vi "BIT2DEC Calculator.vi"() -> ()   [LabVIEW 2022 SP3]
panel:
  out "DEC Data(Result)":dbl
  out "Mantissa Data":dbl
  out "Exponential Data":dbl
  out "Sign Data":dbl
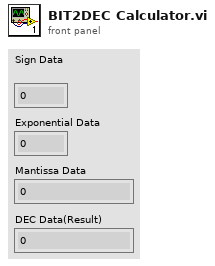
[diagram p1: front panel]
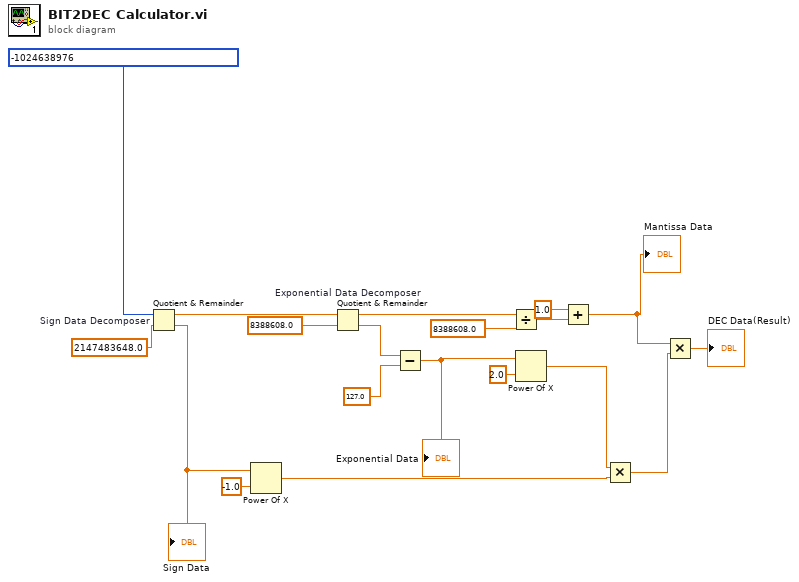
[diagram p0: block diagram]
diagram:
  n1 = Quotient & Remainder "Sign Data Decomposer"(x=-1024638976, y=2147483648.0) -> (x-y*floor(x/y)=w18:dbl, floor(x/y)=w16:dbl)
  "Sign Data" <- w16
  n2 = Power Of X(1:-1.0 ("x"), 2:w16) -> (0:w7:dbl)
  n3 = Quotient & Remainder "Exponential Data Decomposer"(x=w18, y=8388608.0) -> (x-y*floor(x/y)=w11:dbl, floor(x/y)=w13:dbl)
  n4 = Subtract(x=w13, y=127.0) -> (x-y=w9:dbl)
  "Exponential Data" <- w9
  n5 = Divide(x=w11, y=8388608.0) -> (x/y=w3:dbl)
  n6 = Power Of X(1:2.0 ("x"), 2:w9) -> (0:w6:dbl)
  n7 = Add(x=1.0, y=w3) -> (x+y=w1:dbl)
  "Mantissa Data" <- w1
  n8 = Multiply(x=w6, y=w7) -> (x*y=w5:dbl)
  n9 = Multiply(x=w1, y=w5) -> (x*y=→"DEC Data(Result)":dbl)
